vi "Detector ADC.vi"(7 "Address":u16, 8 "Error In":errorcluster, 10 "Detector":u8, 11 "VISA Resource in":refnum<visa-resource-name>) -> (0 "Error Out":errorcluster, 1 "Volatage":dbl[unit] format="%.4f", 2 "ADC Raw":i16, 3 "VISA Resource out":refnum<visa-resource-name>)   [LabVIEW 2014, in "KIT QV.lvlib"]
doc: "Read ADC raw value of selected detector.\n \n<b>Attention:</b> The converion to voltage is estimated, but not calibrated."
uses:
  KIT QV.lvlib
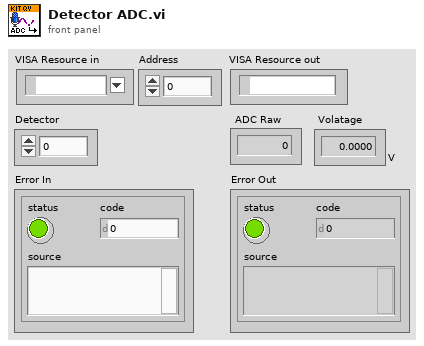
[diagram p1: front panel]
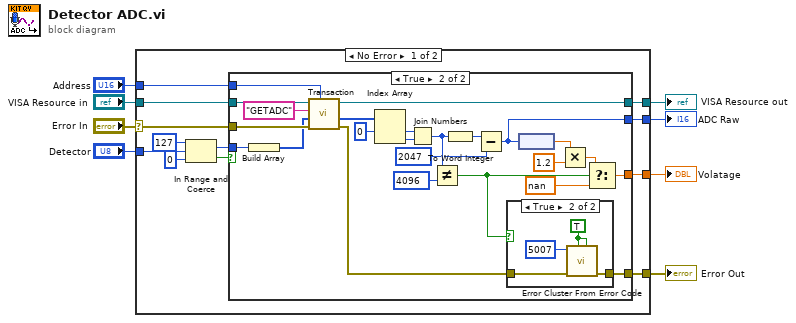
[diagram p0: block diagram]
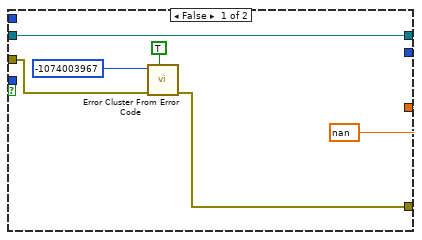
[diagram p2: hidden frame]
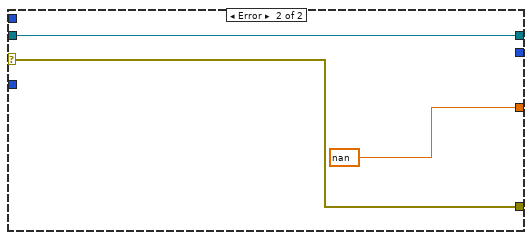
[diagram p4: hidden frame]
diagram:
  n1 = case shown="No Error" "Error In" {
    selector: "Error In" -> [w19 w57]
    tunnel: [w17 w58] -> w8
    tunnel: [w16 w57] -> w7
    tunnel: "VISA Resource in" -> [w20 w58]
    tunnel: "Address" -> [w18 _]
    tunnel: [w15 dbl[unit] nan ("f")] -> w3
    tunnel: [w14 _] -> w2
    tunnel: "Detector" -> [w11 _]
    frame No Error {
      n2 = In Range and Coerce(upper limit=u8 127, x=w11, lower limit=u8 0) -> (coerced(x)=w9:u8, In Range?=w10:bool)
      n3 = case shown="True" w10 {
        tunnel: w20 -> [w26 w50]
        tunnel: w19 -> [w22 w49]
        tunnel: w18 -> [_ w47]
        tunnel: [w26 w46] -> w17
        tunnel: [w21 w27] -> w16
        tunnel: [dbl[unit] nan ("f") w41] -> w15
        tunnel: [_ w32] -> w14
        tunnel: w9 -> [_ w36]
        frame False {
          n4 = call <vilib>:"Error Cluster From Error Code.vi"("show call chain? (False)"=TRUE, "error in (no error)"=w22, "error code (0)"=-1074003967) -> ("error out"=w21:errorcluster)  [unwired: 6 in]
        }
        frame True {
          n5 = Build Array(w36) -> (w35:u8[])
          n6 = call "Transaction.vi"("Address"=w47, "error in (no error)"=w49, "Parameter in"=w35, "Command"="GETADC" ("Reset Command"), "VISA Resource in"=w50) -> ("error out"=w28:errorcluster, "Parameter out"=w45:u8[], "VISA Resource out"=w46:refnum<visa-resource-name>)  [unwired: 4 in]
          n7 = Index Array(array=w45, index #1=0 ("index")) -> (element #1=w43:u8, element #2=w40:u8)  [unwired: 1 in]
          n8 = Join Numbers(hi=w43, lo=w40) -> ((hi.lo)=w34:u16)
          n9 = Not Equal?(x=w34, y=u16 4096) -> (x != y?=w29:bool)
          n10 = To Word Integer(number=w34) -> (16bit integer=w30:i16)
          n11 = Subtract(x=w30, y=i16 2047) -> (x-y=w32:i16)
          n12 = case shown="True" w29 {
            tunnel: w28 -> [w51 w55]
            tunnel: [w51 w54] -> w27
            frame False {
            }
            frame True {
              w52 = TRUE ("show call chain? (False)")
              n13 = call <vilib>:"Error Cluster From Error Code.vi"("is warning? (False)"=w52, "show call chain? (False)"=w52, "error in (no error)"=w55, "error code (0)"=5007) -> ("error out"=w54:errorcluster)  [unwired: 5 in]
            }
          }
          n14 = node(w32) -> (w31:dbl[unit])
          n15 = Multiply(x=w31, y=1.2) -> (x*y=w38:dbl[unit])
          n16 = Select(t=w38, s=w29, f=dbl[unit] nan) -> (s? t:f=w41:dbl[unit])
        }
      }
    }
    frame Error {
    }
  }
  "Error Out" <- w7
  "VISA Resource out" <- w8
  "Volatage" <- w3
  "ADC Raw" <- w2
